vi "WSVCAP SHL Host TL RFFE Write Cycle - Single DUT.vi"(0 "Data Out (Cycle Commands)":string[](array[string]), 5 "Post Command Delay":dbl[](array[numeric]) format="%#.0p s", 11 "error in":errorcluster, 12 "Log (T)":bool=TRUE, 13 "DUT":T1) -> (15 "error out":errorcluster)   [LabVIEW 2012]
uses:
  Type Defs/WSVCAP SHL DUT Number Enum.ctl
  user.lib/Utilities/Type Defs/MISC IO Choice Enum.ctl
panel:
  out "Socket Mask":u64=1 format="%08x"
  out "RFFE Data Out":u8[][](array[numeric]) format="%02x"
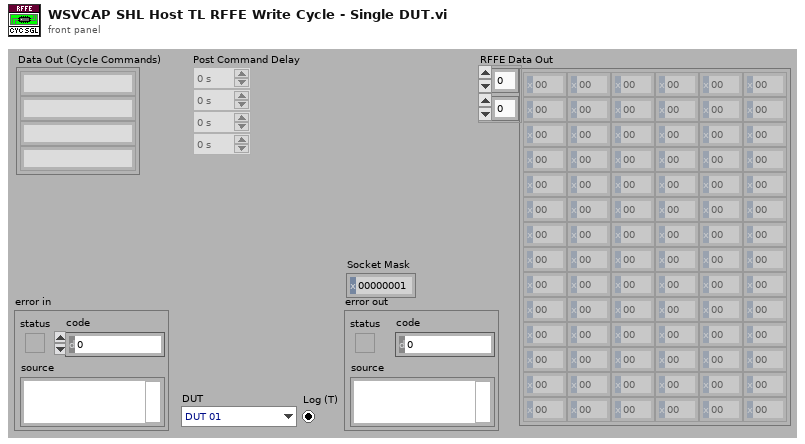
[diagram p1: front panel]
types:
  T1 = typedef "WSVCAP SHL DUT Number Enum.ctl" = enum16{"DUT 01", "DUT 02", "DUT 03", "DUT 04", "DUT 05", "DUT 06", "DUT 07", "DUT 08", "DUT 09", "DUT 10", "DUT 11", "DUT 12", "DUT 13", "DUT 14", "DUT 15", "DUT 16", "DUT 17", "DUT 18", "DUT 19", "DUT 20", "DUT 21", "DUT 22", "DUT 23", "DUT 24", "DUT 25", "DUT 26", "DUT 27", "DUT 28", "DUT 29", "DUT 30", "DUT 31", "DUT 32", "DUT 33", "DUT 34", "DUT 35", "DUT 36"}
  T2 = typedef "MISC IO Choice Enum.ctl" = enum16{"Read", "Write"}
  T3 = typedef "WSVCAP SHL Core System Cluster.ctl" = cluster{"Settings":T4, "FPGA Resource":tag, "Online":bool, "I2C Wait Ticks":u32, "SPI Wait Ticks":u32, "RFFE Wait Ticks":u32}
  T4 = typedef "WSVCAP SHL I2C Settings Cluster.ctl" = cluster{"FPGA Resource Name":string, "I2C Slave Address":u8, "I2C Clock Rate (Hz)":dbl, "SPI Clock Rate (Hz)":dbl, "RFFE Slave Address":u8, "RFFE Clock Rate (Hz)":dbl, "Simulate FPGA":bool, "C1 Cap DAC Default":u8, "C2 Cap DAC Default":u8, "C3 Cap DAC Default":u8}
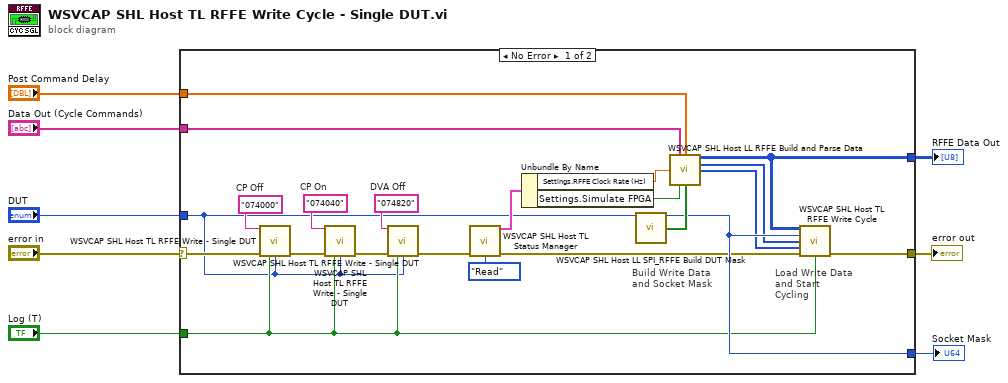
[diagram p0: block diagram]
diagram:
  n1 = case shown="No Error" "error in" {
    selector: "error in" -> [w18 _]
    tunnel: [w26 _] -> w8
    tunnel: [w9 _] -> w6
    tunnel: "DUT" -> [w10 _]
    tunnel: [w29 _] -> w4
    tunnel: "Log (T)" -> [w11 _]
    tunnel: "Post Command Delay" -> [w28 _]
    tunnel: "Data Out (Cycle Commands)" -> [w27 _]
    frame No Error {
      w12 = "074820"  # DVA Off
      w13 = "074040"  # CP On
      w14 = "074000"  # CP Off
      # "Load Write Data and Start Cycling"
      # "Build Write Data and Socket Mask"
      n2 = call "WSVCAP SHL Host TL RFFE Write - Single DUT.vi"("Data Out"=w14, "error in"=w18, "Log (T)"=w11, "DUT"=w10) -> ("error out"=w17:errorcluster)  [unwired: 11 in]
      n3 = call "WSVCAP SHL Host TL RFFE Write - Single DUT.vi"("Data Out"=w13, "error in"=w17, "Log (T)"=w11, "DUT"=w10) -> ("error out"=w16:errorcluster)  [unwired: 11 in]
      n4 = call "WSVCAP SHL Host TL RFFE Write - Single DUT.vi"("Data Out"=w12, "error in"=w16, "Log (T)"=w11, "DUT"=w10) -> ("error out"=w15:errorcluster)  [unwired: 11 in]
      n5 = call "WSVCAP SHL Host TL Status Manager.vi"("error in"=w15, "Operation (Read)"=MISC_IO_Choice_Enum."Read") -> ("System Out"=w23:T3, "error out"=w24:errorcluster)  [unwired: 12 in]
      n6 = Unbundle By Name(w23) -> ("Settings.RFFE Clock Rate (Hz)"=w19:dbl, "Settings.Simulate FPGA"=w22:bool)
      n7 = call "WSVCAP SHL Host LL SPI_RFFE Build DUT Mask.vi"("DUT"=w10) -> ("Socket Mask [U64]"=w29:u64, "DUT Mask"=w30:bool[])  [unwired: 13 in]
      n8 = call "WSVCAP SHL Host LL RFFE Build and Parse Data.vi"("Data Out (Cycle Commands)"=w27, "Post Command Delay"=w28, "Clock Rate (Hz) (Cycle Only)"=w19, "Simulate FPGA (Cycle Only)"=w22, "DUT Mask (All)"=w30) -> ("RFFE Data Out [U8]"=w9:u8[][], "CMD Lengths (Bits)"=w21:u8[], "CMD Delays (Ticks)"=w20:u32[])  [unwired: 7 in, 1 out]
      n9 = call "WSVCAP SHL Host TL RFFE Write Cycle.vi"("RFFE Data Out"=w9, "Socket Mask"=w29, "Cycle CMD Lengths (bits)"=w21, "Cycle CMD Delay (ticks)"=w20, "error in"=w24, "Log (T)"=w11) -> ("error out"=w26:errorcluster)  [unwired: 9 in]
    }
    frame Error {
    }
  }
  "error out" <- w8
  "RFFE Data Out" <- w6
  "Socket Mask" <- w4
